vi "Operator Dialog for Key Press Base.vi"() -> ()   [LabVIEW 2024, in "Vehicle.lvclass"]
uses:
  Vehicle.lvclass
  Vehicle.lvclass/Vehicle.ctl
panel:
  in  "Boolean":bool
  # "Press KeyFob Base"
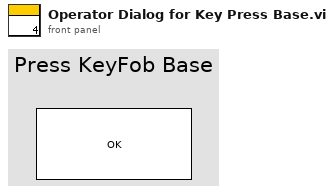
[diagram p1: front panel]
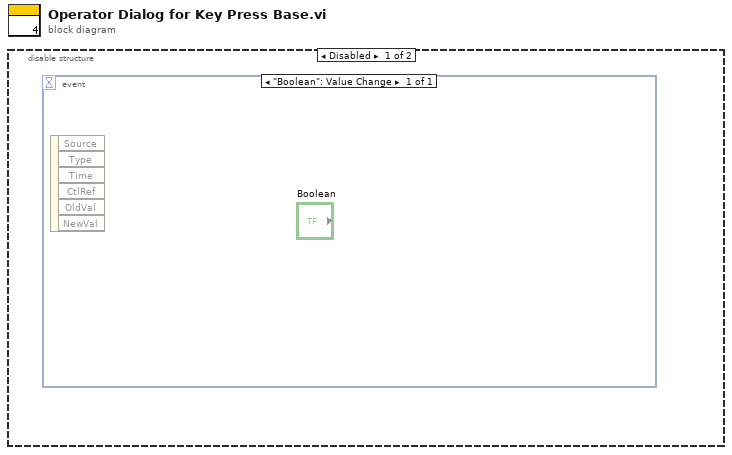
[diagram p0: block diagram]
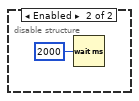
[diagram p2: hidden frame]
diagram:
  n1 = disable-structure shown="Disabled" {
    frame Disabled {
      n2 = event shown="[0] \"Boolean\": Value Change" {
        selector: _ -> [_]
        dyn-events: _ -> [_]
        timeout: _ -> [_]
        event "Boolean": Value Change {
          n3 = event-data() -> ()  [unwired: 1 in, 6 out]
        }
      }
    }
    frame Enabled {
      n4 = Wait (ms)(milliseconds to wait=u32 2000) -> ()  [unwired: 1 out]
    }
  }
